vi "Binario.vi"(8 "error in (no error)":errorcluster, 10 "signal out":waveform(dbl), 11 "Binary in":refnum<class "Binary.lvclass">) -> (0 "error out":errorcluster, 3 "Loggin out":refnum<class "Loggin.lvclass">)   [LabVIEW 2020, in "Binary.lvlib" / "Binary.lvclass"]
uses:
  Binary.lvclass
  C:/Users/Ceci Saldivar/Desktop/ceci/7mo semestre/Henry/Actor-Tarea-10-12-2020/Loggin/Loggin/Loggin.lvclass
  Loggin/Loggin/Loggin.lvclass
  Loggin/Loggin/Loggin.lvclass/Loggin.ctl
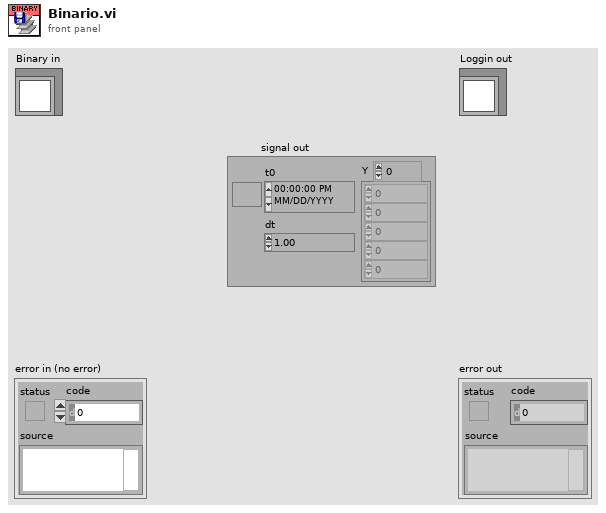
[diagram p1: front panel]
types:
  T1 = enum16{"open", "replace", "create", "open or create", "replace or create", "replace or create with confirmation"}
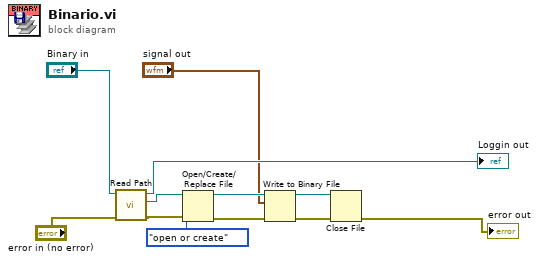
[diagram p0: block diagram]
diagram:
  n1 = call "Read Path.vi"("error in (no error)"="error in (no error)", "Loggin in"="Binary in") -> ("error out"=w5:errorcluster, "Path"=w3:path, "Loggin out"=→"Loggin out":refnum<class "Binary.lvclass">)  [unwired: 7 in]
  n2 = Open/Create/Replace File(file path (use dialog)=w3, error in=w5, operation (0:open)=T1."open or create") -> (refnum out=w9:refnum<file>, error out=w12:errorcluster)  [unwired: 3 in, 1 out]
  n3 = Write to Binary File(file (use dialog)=w9, data="signal out", error in=w12) -> (refnum out=w8:refnum<file>, error out=w11:errorcluster)  [unwired: 3 in, 1 out]
  n4 = Close File(refnum=w8, error in=w11) -> (error out=→"error out":errorcluster)  [unwired: 1 out]
